vi "Turret Structure.vi"(0 "AIDeviceRef":T1, 1 "Raw Turret":dbl, 2 "Left":dbl=4.5, 3 "Right":dbl=0.85, 5 "Turret Case":i32, 7 "Home Speed":dbl=1.0, 9 "Home postion":dbl, 11 "error in (no error)":errorcluster, 12 "Auton Right":dbl) -> (6 "Turret Output":dbl, 15 "Turret Case Output":dbl)   [LabVIEW 2011]
uses:
  <vilib>/Rock Robotics/WPI/AnalogChannel/WPI_AnalogChannelDevRef.ctl
  <vilib>/Rock Robotics/SystemInterfaces/Typedef/FPGA_TypedefAnalogModule.ctl
  <vilib>/Rock Robotics/SystemInterfaces/AI/FPGA_AIChannel.ctl
  Robot Global Data.vi
  <vilib>/addons/control/pid/pid.llb/PID (DBL).vi
  <vilib>/addons/control/pid/NI_PID_pid.lvlib
panel:
  in  "-1/1 per degree":dbl=0.05
  in  "Volts per degree":dbl=0.0166666666666667
  in  "PID Gains":T4={"proportional gain (Kc)"=1.0, "integral time (Ti, min)"=0.01, "derivative time (Td, min)"=0.0} {"derivative time (Td, min)" format="%.3f"; "integral time (Ti, min)" format="%.3f"; "proportional gain (Kc)" format="%.3f"}
  out "Waveform Chart":dynamicdata(graph)
  in  "PID Enable":bool
  # "Bring from Right to Left"
  # "Right Joystick moves Left"
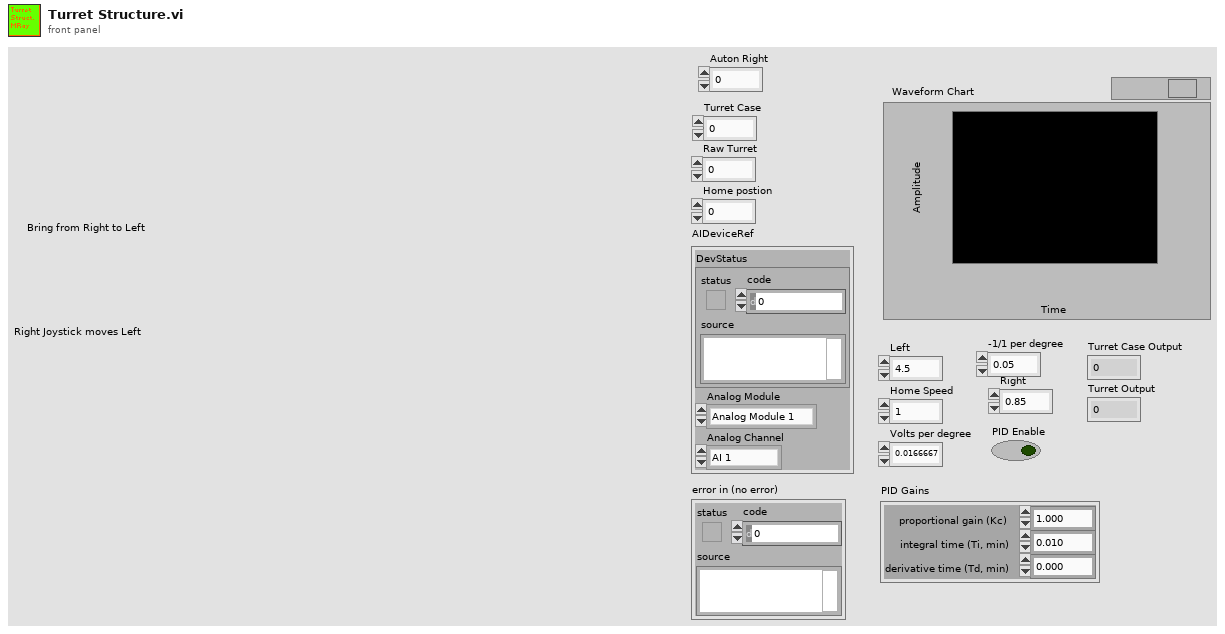
[diagram p1: front panel]
types:
  T1 = typedef "WPI_AnalogChannelDevRef.ctl" = cluster{"DevStatus":errorcluster, "Analog Module":T2, "Analog Channel":T3}
  T2 = typedef "FPGA_TypedefAnalogModule.ctl" = enum16{"Analog Module 1", "Analog Module 2"}
  T3 = typedef "FPGA_AIChannel.ctl" = enum8{"AI 1", "AI 2", "AI 3", "AI 4", "AI 5", "AI 6", "AI 7", "AI 8", "Invalid"}
  T4 = cluster{"proportional gain (Kc)":dbl, "integral time (Ti, min)":dbl, "derivative time (Td, min)":dbl}
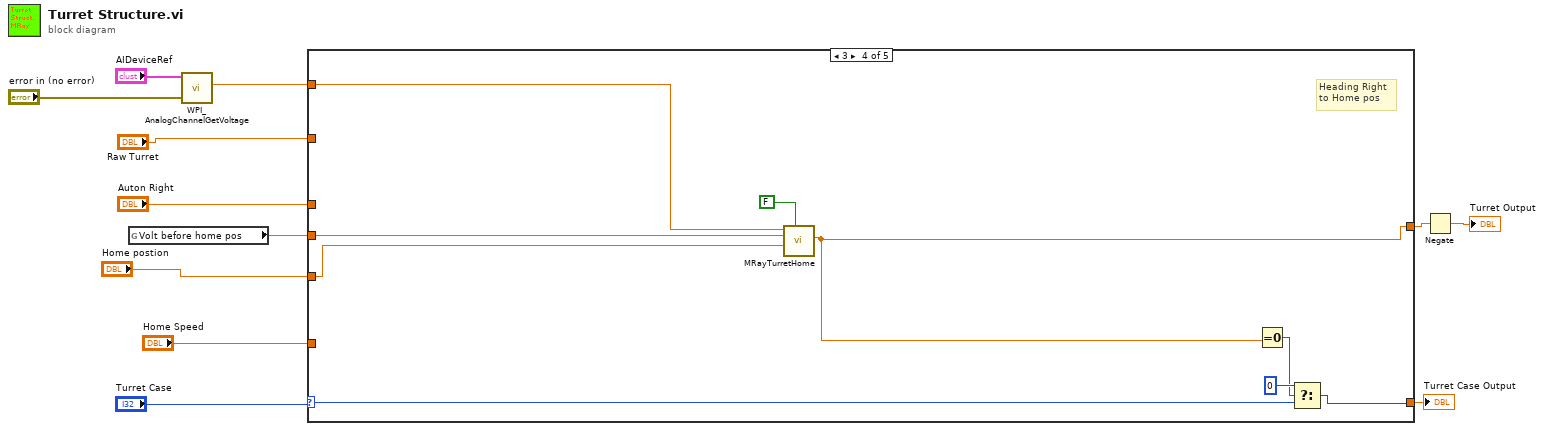
[diagram p0: block diagram]
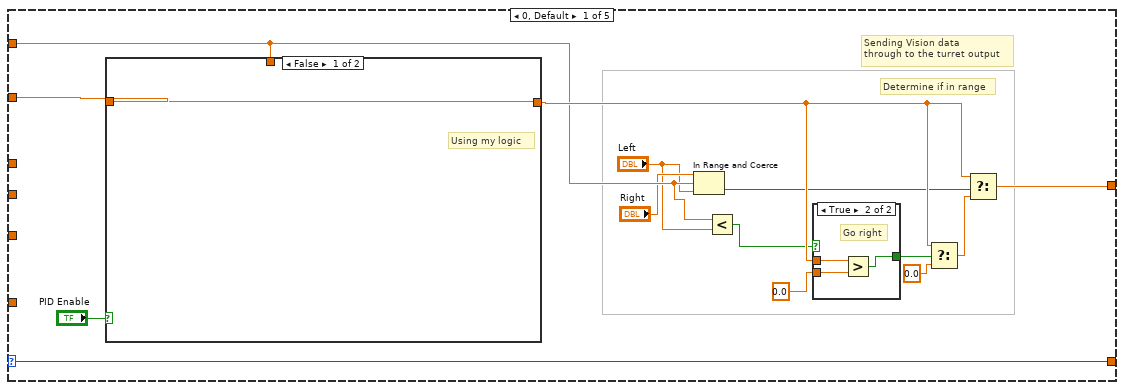
[diagram p2: hidden frame]
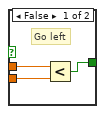
[diagram p3: hidden frame]
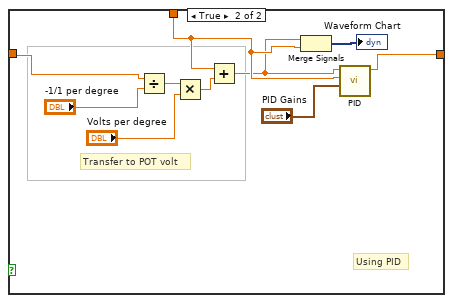
[diagram p4: hidden frame]
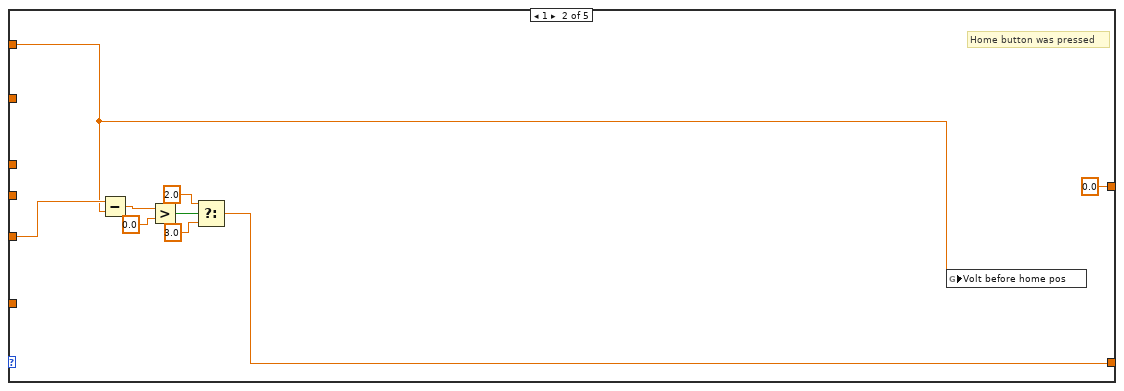
[diagram p5: hidden frame]
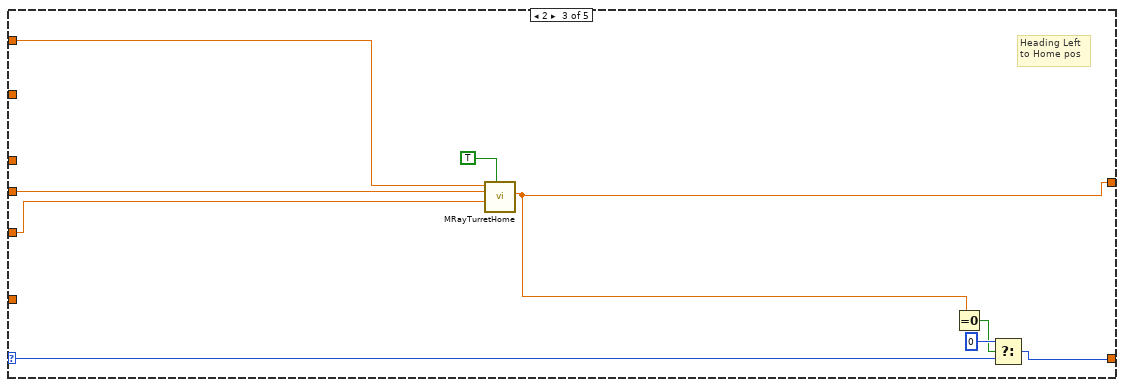
[diagram p6: hidden frame]
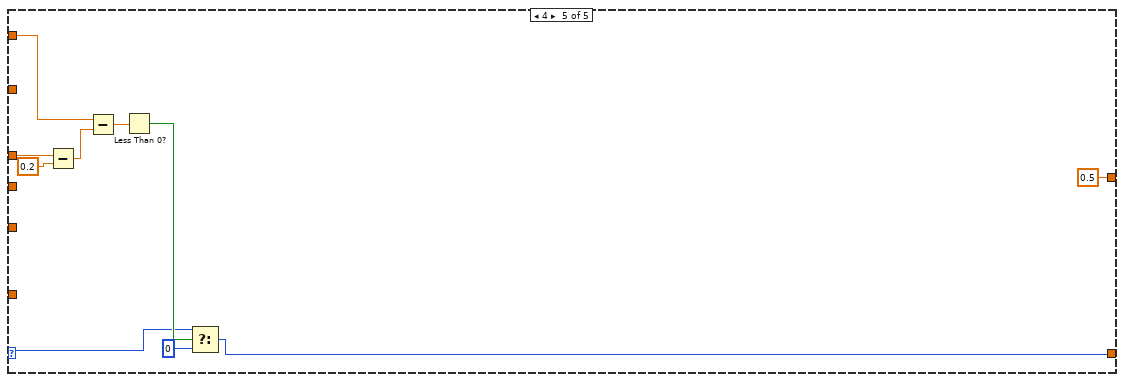
[diagram p7: hidden frame]
diagram:
  n1 = global read "Robot Global Data.vi" "Volt before home pos"() -> (w1:dbl)
  n2 = call <vilib>:"WPI_AnalogChannelGetVoltage.vi"("error in (no error)"="error in (no error)", "AIDeviceRef"="AIDeviceRef") -> ("Voltage"=w12:dbl)  [unwired: 7 in, 2 out]
  n3 = case shown="3" "Turret Case" {
    selector: "Turret Case" -> [w18 _ w61 w69 w77]
    tunnel: w12 -> [w17 w44 w58 w66 w80]
    tunnel: "Raw Turret" -> [w25 _ _ _ _]
    tunnel: [w19 0.0 ("Home Speed 2") w53 w63 0.5 ("Home Speed")] -> w4
    tunnel: "Home postion" -> [_ w49 w59 w67 _]
    tunnel: [w18 w48 w60 w68 w75] -> w5
    tunnel: "Home Speed" -> [_ _ _ _ _]
    tunnel: "Auton Right" -> [_ _ _ _ w73]
    tunnel: w1 -> [_ _ w56 w64 _]
    frame 0, Default {
      # "Determine if in range"
      # "Sending Vision data\nthrough to the turret output"
      n4 = case shown="False" "PID Enable" {
        tunnel: w25 -> [w33 w42]
        tunnel: [w33 w37] -> w21
        tunnel: w17 -> [_ w35]
        frame False {
          # "Using my logic"
        }
        frame True {
          # "Transfer to POT volt"
          # "Using PID"
          n5 = Divide(x=w42, y="-1/1 per degree") -> (x/y=w41:dbl)
          n6 = Multiply(x=w41, y="Volts per degree") -> (x*y=w39:dbl)
          n7 = Add(x=w35, y=w39) -> (x+y=w34:dbl)
          n8 = Merge Signals(w34, w35) -> (→"Waveform Chart":dynamicdata)
          n9 = call-poly <vilib>:"PID.vi"("PID gains"="PID Gains", "process variable"=w35, "setpoint"=w34) -> ("output"=w37:dbl)  [unwired: 7 in, 1 out]
        }
      }
      n10 = In Range and Coerce(upper limit="Right", x=w17, lower limit="Left") -> (In Range?=w16:bool)  [unwired: 1 out]
      n11 = Less?(x=w17, y="Left") -> (x < y?=w13:bool)
      n12 = case shown="True" w13 {
        tunnel: 0.0 -> [w28 w32]
        tunnel: [w27 w31] -> w22
        tunnel: w21 -> [w29 w30]
        frame False {
          # "Go left"
          n13 = Less?(x=w29, y=w28) -> (x < y?=w27:bool)
        }
        frame True {
          # "Go right"
          n14 = Greater?(x=w30, y=w32) -> (0:w31:bool)
        }
      }
      n15 = Select(t=w21, s=w22, f=0.0) -> (s? t:f=w20:dbl)
      n16 = Select(t=w21, s=w16, f=w20) -> (s? t:f=w19:dbl)
    }
    frame 1 {
      # "Home button was pressed"
      n17 = Subtract(x=w49, y=w44) -> (x-y=w50:dbl)
      n18 = Greater?(x=w50, y=0.0) -> (0:w52:bool)
      n19 = Select(t=2.0, s=w52, f=3.0) -> (s? t:f=w48:dbl)
      n20 = global write "Robot Global Data.vi" "Volt before home pos"(w44) -> ()
    }
    frame 2 {
      # "Heading Left\nto Home pos"
      n21 = call "MRayTurretHome.vi"("Left to right"=TRUE, "Home volt"=w59, "Volt at start"=w56, "Turret POT volt"=w58) -> ("Turret Output"=w53:dbl)  [unwired: 7 in]
      n22 = Equal To 0?(x=w53) -> (x = 0?=w54:bool)
      n23 = Select(t=0, s=w54, f=w61) -> (s? t:f=w60:i32)
    }
    frame 3 {
      # "Heading Right\nto Home pos"
      n24 = call "MRayTurretHome.vi"("Left to right"=FALSE, "Home volt"=w67, "Volt at start"=w64, "Turret POT volt"=w66) -> ("Turret Output"=w63:dbl)  [unwired: 7 in]
      n25 = Equal To 0?(x=w63) -> (x = 0?=w62:bool)
      n26 = Select(t=0, s=w62, f=w69) -> (s? t:f=w68:i32)
    }
    frame 4 {
      n27 = Subtract(x=w73, y=0.2) -> (x-y=w71:dbl)
      n28 = Subtract(x=w80, y=w71) -> (x-y=w79:dbl)
      n29 = Less Than 0?(x=w79) -> (x < 0?=w78:bool)
      n30 = Select(t=w77, s=w78, f=0) -> (s? t:f=w75:i32)
    }
  }
  "Turret Case Output" <- w5
  n31 = Negate(x=w4) -> (-x=→"Turret Output":dbl)
